vi "Initialize MeasurementLink Session.vi"(7 "remote connection options":T2, 8 "error in":errorcluster, 9 "initialize and close session behavior":T1, 10 "session initialization parameters":T3, 11 "session factory in":refnum<class "Session Factory.lvclass">) -> (0 "error out":errorcluster, 2 "session out":variant, 3 "session factory out":refnum<class "Session Factory.lvclass">)   [LabVIEW 2025, in "Session Management flexrio 148x.lvlib" / "Session Factory.lvclass"]
doc: "Creates a new session using the provided <b>session initialization parameters</b>. If the session represents a remote session, <b>initialize and close session behavior</b> determines whether creating the local session creates a new session on the server or attaches to an existing session on the server."
uses:
  Session Factory.lvclass
  <vilib>/Plug-In SDKs/Sessions/Instrument/ISession Factory/Remote Connection Options.ctl
  <vilib>/Plug-In SDKs/Sessions/Instrument/ISession Factory/ISession Factory.lvclass
  <vilib>/Plug-In SDKs/Sessions/Instrument/ISession Factory/Initialize and Close Session Behavior.ctl
  <vilib>/Plug-In SDKs/Sessions/Instrument/ISession Factory/Session Initialization Parameters.ctl
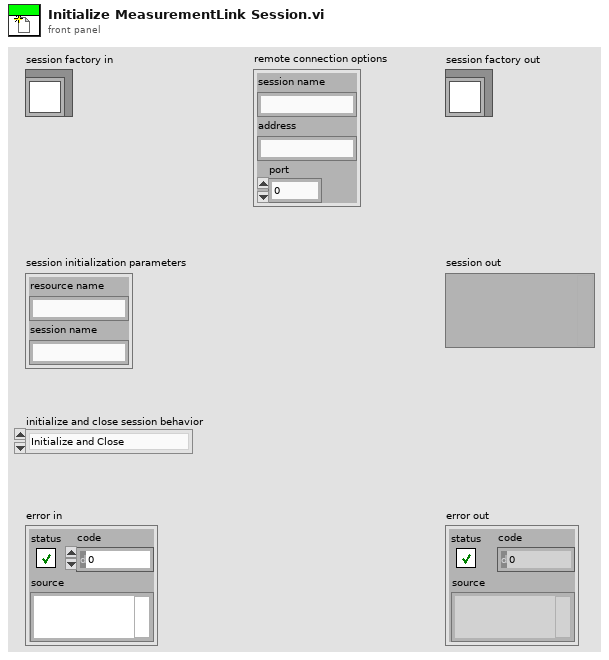
[diagram p1: front panel]
types:
  T1 = typedef "NI Session Management Instrument.lvlib/ISession Factory.lvclass/Initialize and Close Session Behavior.ctl" = enum16{"Initialize and Close", "Attach and Detach", "Initialize and Detach", "Attach and Close"}
  T2 = typedef "NI Session Management Instrument.lvlib/ISession Factory.lvclass/Remote Connection Options.ctl" = cluster{"session name":string, "address":string, "port":u32}
  T3 = typedef "NI Session Management Instrument.lvlib/ISession Factory.lvclass/Session Initialization Parameters.ctl" = cluster{"resource name":string, "session name":string}
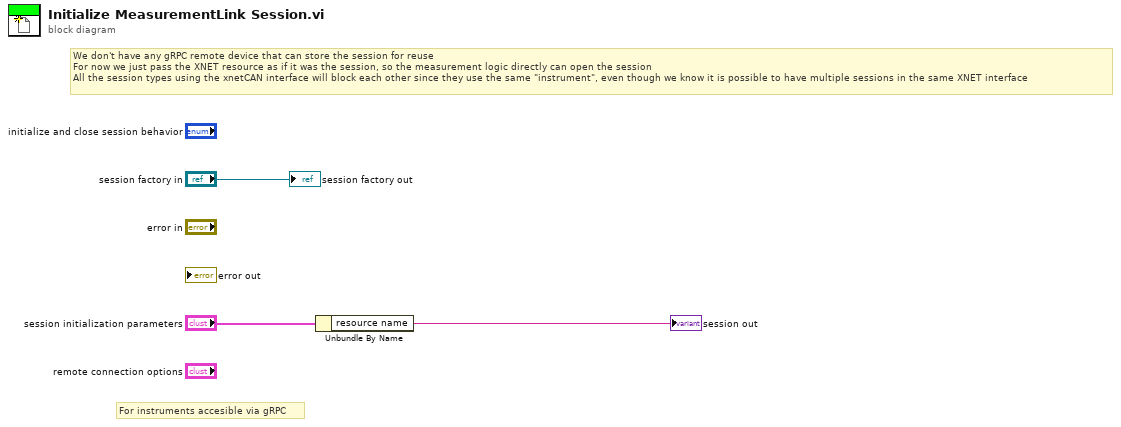
[diagram p0: block diagram]
diagram:
  # "We don't have any gRPC remote device that can store the session for reuse\nFor now we just pass the XNET resource as if it was the session, so the measurement logic directly can open the session\nAll the session types using the xnetCAN interface will block each other since they use the same \"instrument\", even though we know it is possible to have multiple sessions in the same XNET interface"
  # "For instruments accesible via gRPC"
  n1 = Unbundle By Name("session initialization parameters") -> ("resource name"=→"session out":string)
  "session factory out" <- "session factory in"
